vi "Eval.vi"(8 "error in (no error)":errorcluster, 11 "muExpr in":refnum<class "mupExpr.lvclass">) -> (0 "error out":errorcluster, 2 "Result":dbl format="%#_13g", 3 "muExpr out":refnum<class "mupExpr.lvclass">)   [LabVIEW 2015, in "mupExpr.lvclass"]
uses:
  mupExpr.lvclass
  mupExpr.lvclass/mupExpr.ctl
  mupLib/mupCheckError.vi
  mupLib/mupLibPath.vi
  mupLib/mupLib.lvlib
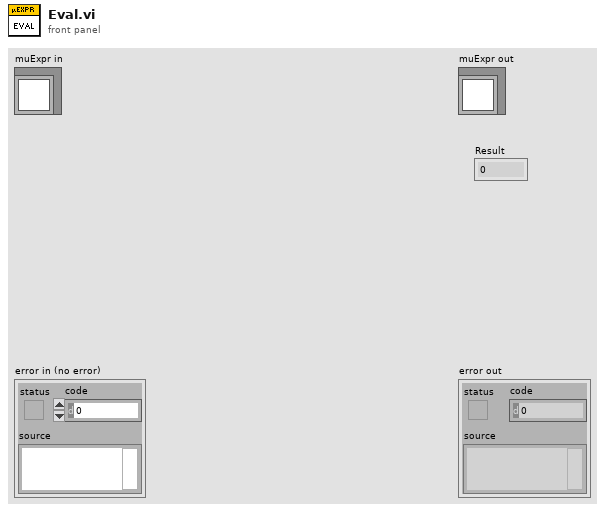
[diagram p1: front panel]
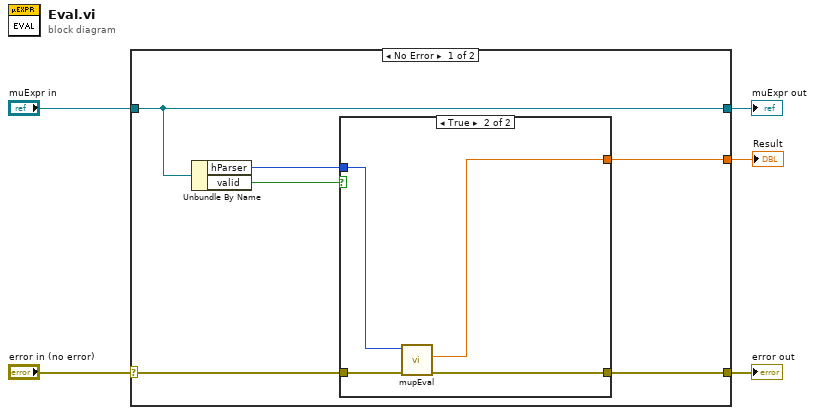
[diagram p0: block diagram]
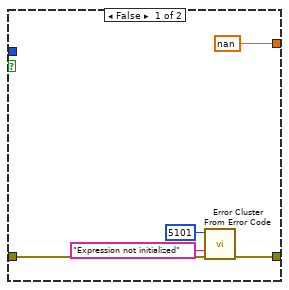
[diagram p2: hidden frame]
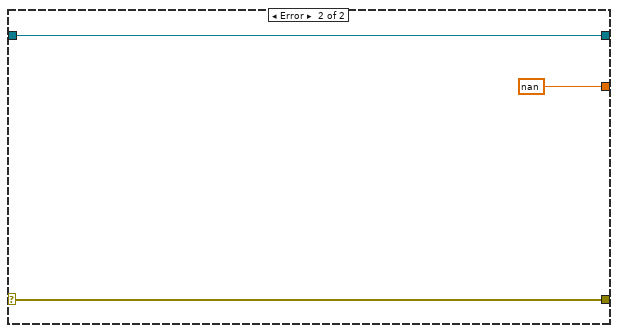
[diagram p3: hidden frame]
diagram:
  n1 = case shown="No Error" "error in (no error)" {
    selector: "error in (no error)" -> [w10 w23]
    tunnel: [w9 w23] -> w4
    tunnel: [w11 w22] -> w2
    tunnel: "muExpr in" -> [w11 w22]
    tunnel: [w8 nan ("return type")] -> w1
    frame No Error {
      n2 = Unbundle By Name(w11) -> ("hParser"=w7:u64, "valid"=w6:bool)
      n3 = case shown="True" w6 {
        tunnel: w10 -> [w15 w19]
        tunnel: [w14 w17] -> w9
        tunnel: [nan ("return type") w18] -> w8
        tunnel: w7 -> [_ w20]
        frame False {
          n4 = call <vilib>:"Error Cluster From Error Code.vi"("error in (no error)"=w15, "error message (\"\")"="Expression not initialized" ("error message (\"\")"), "error code (0)"=5101) -> ("error out"=w14:errorcluster)  [unwired: 6 in]
        }
        frame True {
          n5 = call "mupEval.vi"("error in (no error)"=w19, "hParser in"=w20) -> ("error out"=w17:errorcluster, "result"=w18:dbl)  [unwired: 7 in, 1 out]
        }
      }
    }
    frame Error {
    }
  }
  "error out" <- w4
  "muExpr out" <- w2
  "Result" <- w1
